vi "CPP-GRCserver.vi"(4 "minFlowrate (l/min)":dbl format="%.2f", 5 "Pressure channel":string, 6 "maxFlowrate (l/min)":dbl format="%.2f", 7 "Temperature channel":string, 8 "C:Dem(%)":dbl caption="C:Dem(%) (0)" min=0.0 max=100.0 step=1.0 format="%.2f", 9 "Gas Release System":string, 10 "Q[Total]:Dem(l/min)":dbl caption="Q[Total]:Dem(l/min) (0)" format="%.2f", 11 "Mode":T1=enum."Close All MFCs" caption="Mode (CloseAll)") -> (0 "errorString":string, 1 "infoString":string, 3 "watchChannels":string[](array[string]))   [LabVIEW 2021]
uses:
  Sub VI's/Gas management/CPP/AalborgServerModes.ctl
  Sub VI's/Gas management/CPP/AalborgServerData.ctl
  Sub VI's/Gas management/CPP/MFCdescription.ctl
  Sub VI's/Gas management/CPP/MFCcapability.ctl
  Sub VI's/Gas management/CPP/AalborgServerControlBus.ctl
  Sub VI's/Gas management/CPP/AalborgServerStates.ctl
  ADAM Client/Sub VIs/ADAM Controls/Channel_State.ctl
  ADAM Client/Sub VIs/ADAM Controls/Update_scan_value.ctl
  Anemometry/Anemometry Sub Vis/Controls/GasCombo.ctl
  f0e89fe8-b597-9c4c-bd9e-b7a5d13a6cec.vi
panel:
  in  "Tab Control":enum32{"I/O", "Control", "Data"}(tab)
  out "callNum":i32
  in  "idealSPFraction":dbl=0.95 format="%#_13g"
  out "Press:(mBar)":dbl
  out "Temp:(C)":dbl
  out "C2H6 massflow demand":dbl format="%#_g g/min"
  out "N2 massflow demand":dbl format="%#_g g/min"
  out "C2H6 flowrate demand":dbl format="%#_g l/min"
  out "N2 flowrate demand":dbl format="%#_g l/min"
  out "runTime(s)":dbl
  out "ControlBus":T2={"ActionPath"=[enum."ComputeFlowrates", enum."ADAMiseDemands", enum."ListMFCchannels", enum."ChooseMFCs", enum."CalculateSetpoints", enum."ExecuteSetpoints", enum."Summarise"], "step"=0, "Done?"=FALSE, "Messages"="", "deltaQ"=0.0, "deltaC"=0.0}
  out "DataBus":T4 {"RhoTrace" format="%.3gg/l"; "RhoCarrier" format="%.3gg/l"; "InactiveC2H6MFCs"."mDot" format="%_4g"; "InactiveC2H6MFCs"."Setpoint" format="%.2g"; "InactiveC2H6MFCs"."MFCcapability"."MaxMdot" format="%_4g"; "InactiveC2H6MFCs"."MFCcapability"."MinMdot" format="%_4g"; "ActiveC2H6MFCs"."mDot" format="%_4g"; "ActiveC2H6MFCs"."Setpoint" format="%.2g"; "ActiveC2H6MFCs"."MFCcapability"."MaxMdot" format="%_4g"; "ActiveC2H6MFCs"."MFCcapability"."MinMdot" format="%_4g"; "InactiveN2MFCs"."mDot" format="%_4g"; "InactiveN2MFCs"."Setpoint" format="%.2g"; "InactiveN2MFCs"."MFCcapability"."MaxMdot" format="%_4g"; "InactiveN2MFCs"."MFCcapability"."MinMdot" format="%_4g"; "ActiveN2MFCs"."mDot" format="%_4g"; "ActiveN2MFCs"."Setpoint" format="%.2g"; "ActiveN2MFCs"."MFCcapability"."MaxMdot" format="%_4g"; "ActiveN2MFCs"."MFCcapability"."MinMdot" format="%_4g"; "C2H6MFCs"."mDot" format="%_4g"; "C2H6MFCs"."Setpoint" format="%.2g"; "C2H6MFCs"."MFCcapability"."MaxMdot" format="%_4g"; "C2H6MFCs"."MFCcapability"."MinMdot" format="%_4g"; "N2MFCs"."mDot" format="%_4g"; "N2MFCs"."Setpoint" format="%.2g"; "N2MFCs"."MFCcapability"."MaxMdot" format="%_4g"; "N2MFCs"."MFCcapability"."MinMdot" format="%_4g"; "QdemCarrier" format="%.2pl/min"; "QdemTrace" format="%.2pl/min"; "MdotCarrier" format="%_4pg/min"; "MdotTrace" format="%_4pg/min"; "releaseTemp" format="%#_gC"; "releasePress" format="%#_gmBar"}
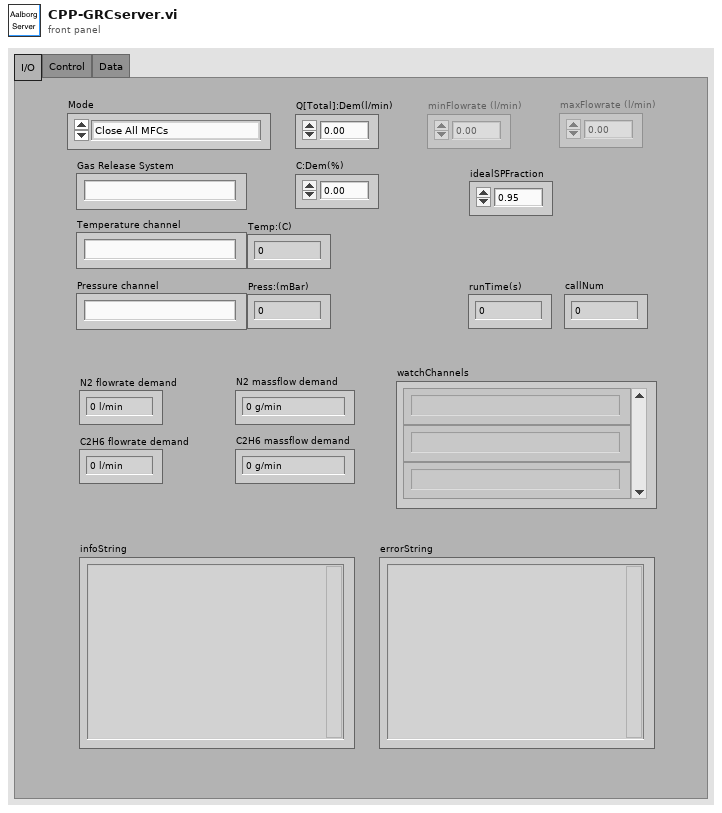
[diagram p1: front panel]
types:
  T1 = typedef "AalborgServerModes.ctl" = enum16{"Set Flows", "Check Flows Are Achievable", "Close All MFCs"}
  T2 = typedef "AalborgServerControlBus.ctl" = cluster{"ActionPath":T3[], "step":i32, "Done?":bool, "Messages":string, "deltaQ":dbl, "deltaC":dbl}
  T3 = typedef "AalborgServerStates.ctl" = enum16{"Initialise", "Supervise", "WhatNext", "ComputeFlowrates", "ADAMiseDemands", "ListMFCchannels", "ChooseMFCs", "CalculateSetpoints", "ExecuteSetpoints", "SetScanRates", "CloseAll", "Summarise"}
  T4 = typedef "AalborgServerData.ctl" = cluster{"releaseTemp":dbl, "releasePress":dbl, "QdemCarrier":dbl, "QdemTrace":dbl, "MdotCarrier":dbl, "MdotCarrierMin":dbl, "MdotCarrierMax":dbl, "MdotTrace":dbl, "MdotTraceMin":dbl, "MdotTraceMax":dbl, "N2MFCs":T5[], "C2H6MFCs":T5[], "CarrierOffIdeal":dbl, "TraceOffIdeal":dbl, "ActiveN2MFCs":T5[], "InactiveN2MFCs":T5[], "ActiveC2H6MFCs":T5[], "InactiveC2H6MFCs":T5[], "RhoCarrier":dbl, "RhoTrace":dbl}
  T5 = typedef "MFCdescription.ctl" = cluster{"BaseName":string, "MFCcalibration":cluster{"Y(100)":dbl, "Y(0)":dbl, "SPmin(%)":dbl, "SPmax(%)":dbl}, "MFCcapability":T6, "InUse?":bool, "Setpoint":dbl, "mDot":dbl}
  T6 = typedef "MFCcapability.ctl" = cluster{"Gas":string, "MinMdot":dbl, "MaxMdot":dbl}
  T7 = typedef "Channel_State.ctl" = enum16{"On", "Off", "Always On", "Always Off"}
  T8 = typedef "GasCombo.ctl" = string
  T9 = typedef "Update_scan_value.ctl" = cluster{"Channel Name":string, "New Value":dbl, "!Auto_Off":bool}
  T10 = typedef "Ch_description_ADAM.ctl" = cluster{"Ch Name":string, "Type":T11, "Function":T12, "Ch State":T7, "Calibration type":T13, "A":dbl, "B":dbl, "C":dbl, "D":dbl, "Comments":string, "Address":T14, "String":string, "Duty":u16}
  T11 = typedef "Module_type_ADAM.ctl" = string
  T12 = typedef "Function_ADAM.ctl" = enum16{"Analogue Input", "Digital Input", "Event counter", "Event rate", "Analogue Output", "Digital Output", "Relay Output"}
  T13 = typedef "Calib_type_ADAM.ctl" = string
  T14 = typedef "Address.ctl" = cluster{"Main":i32, "Ch.":i32, "Sub":i32, "Port Name":string}
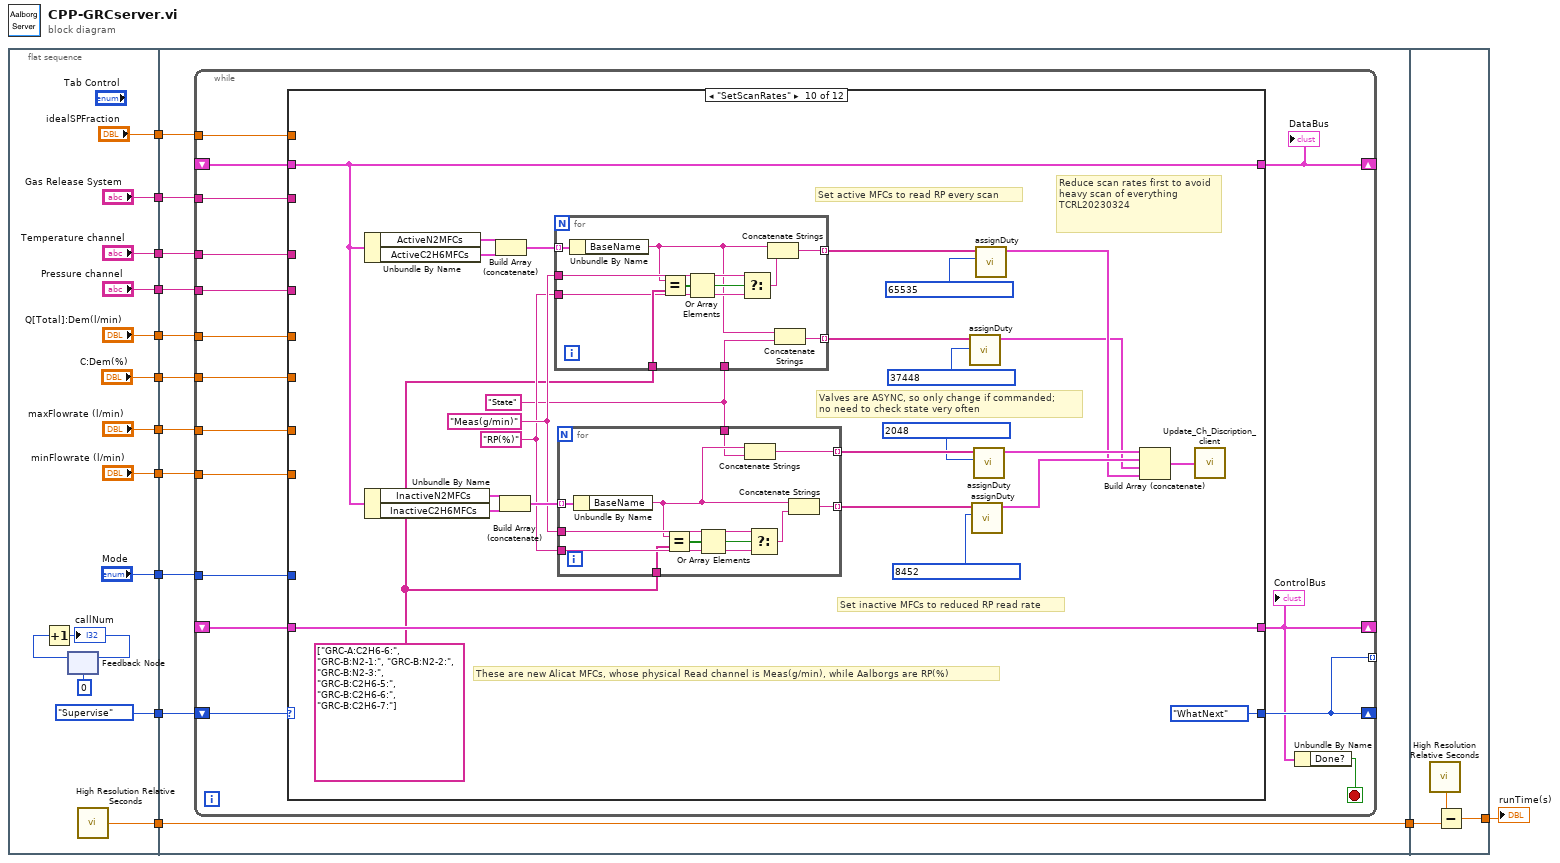
[diagram p0: block diagram]
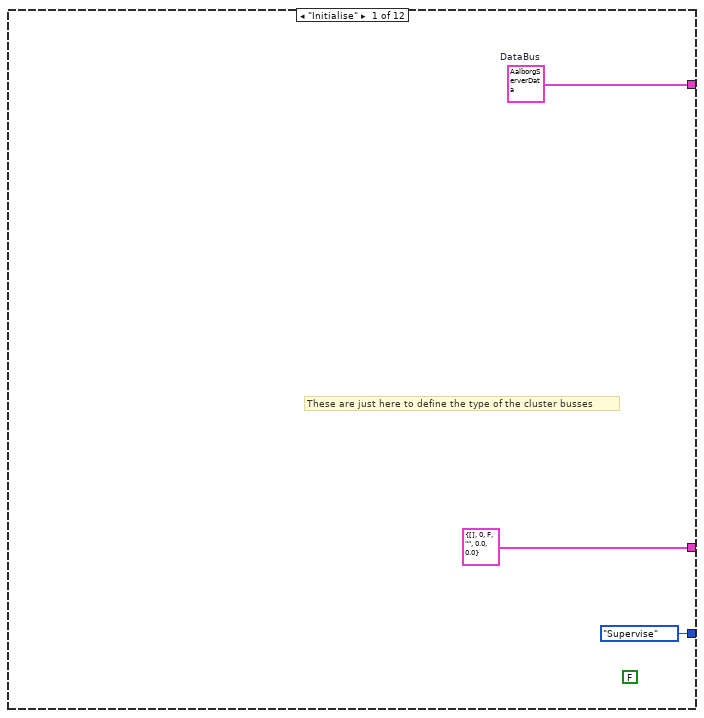
[diagram p2: hidden frame]
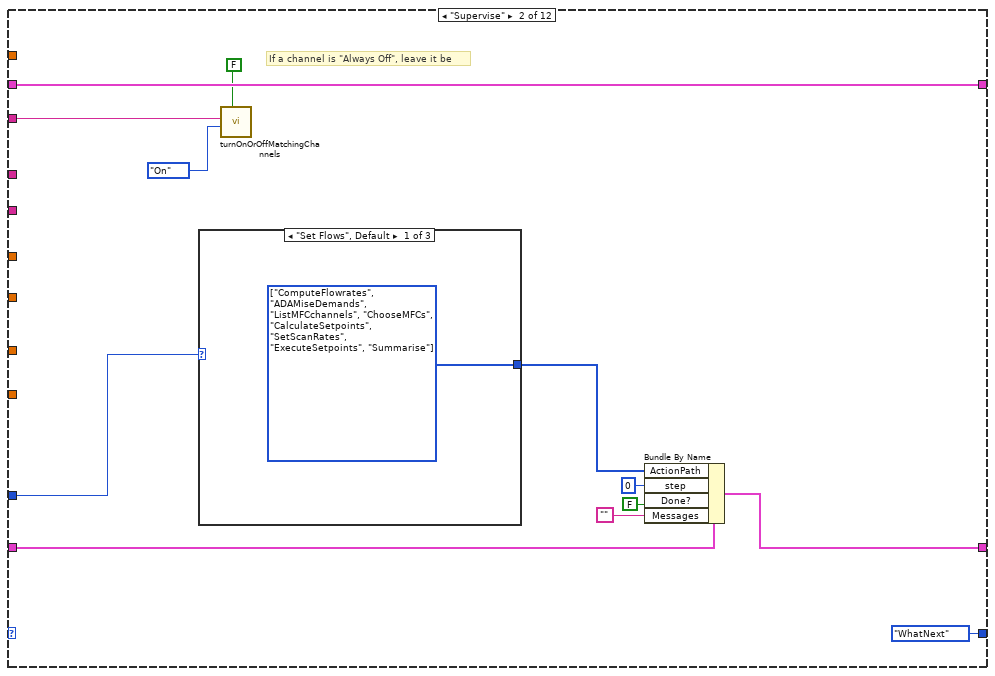
[diagram p3: hidden frame]
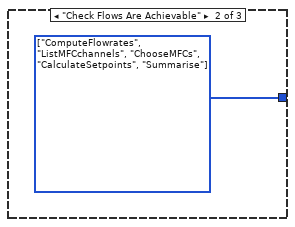
[diagram p4: hidden frame]
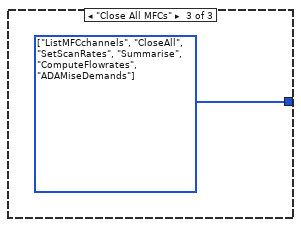
[diagram p5: hidden frame]
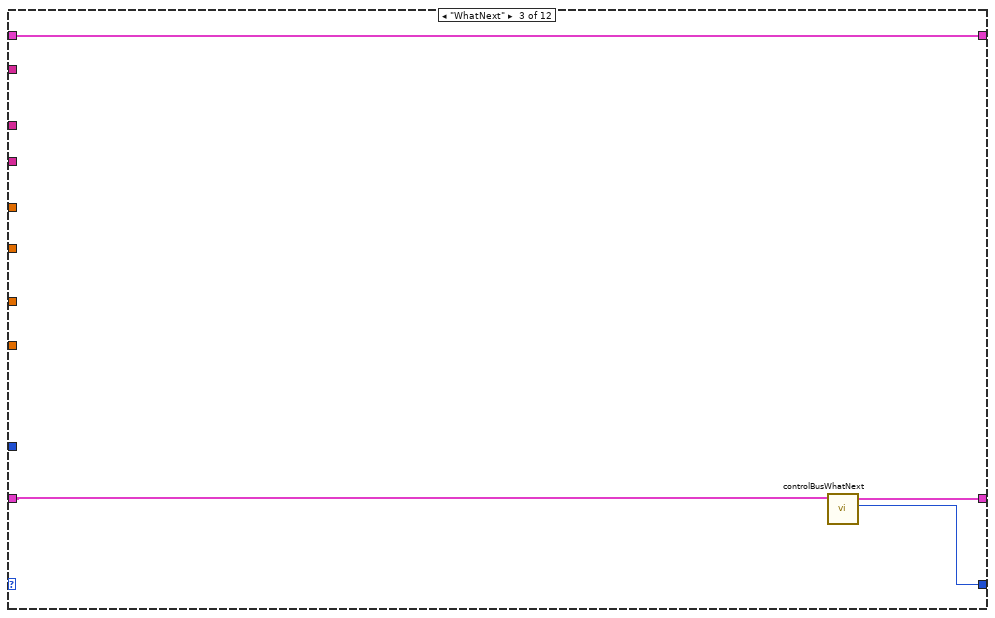
[diagram p6: hidden frame]
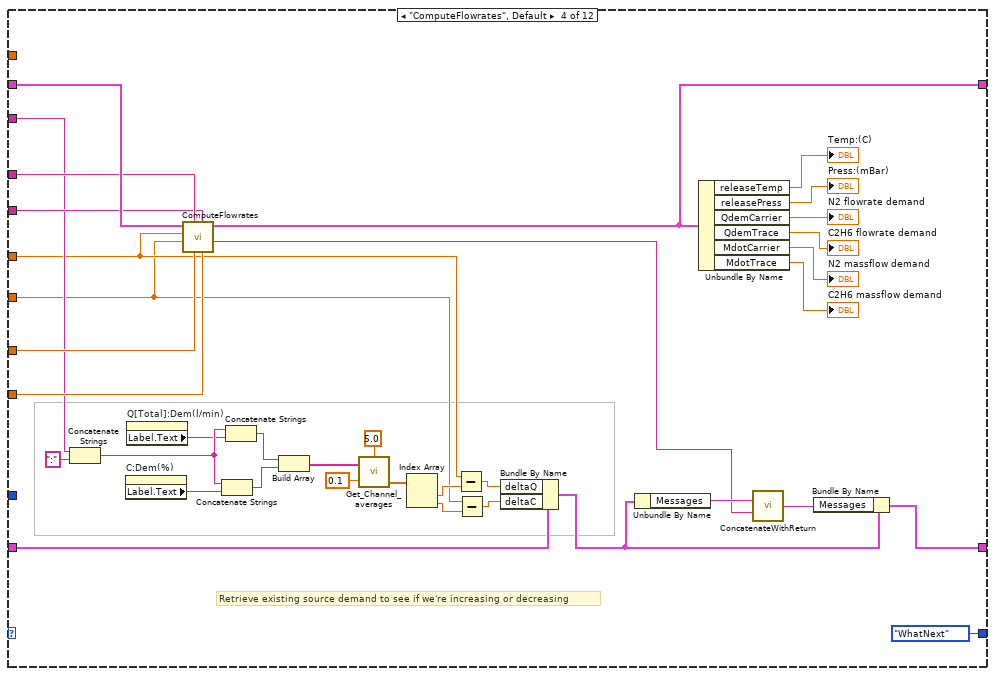
[diagram p7: hidden frame]
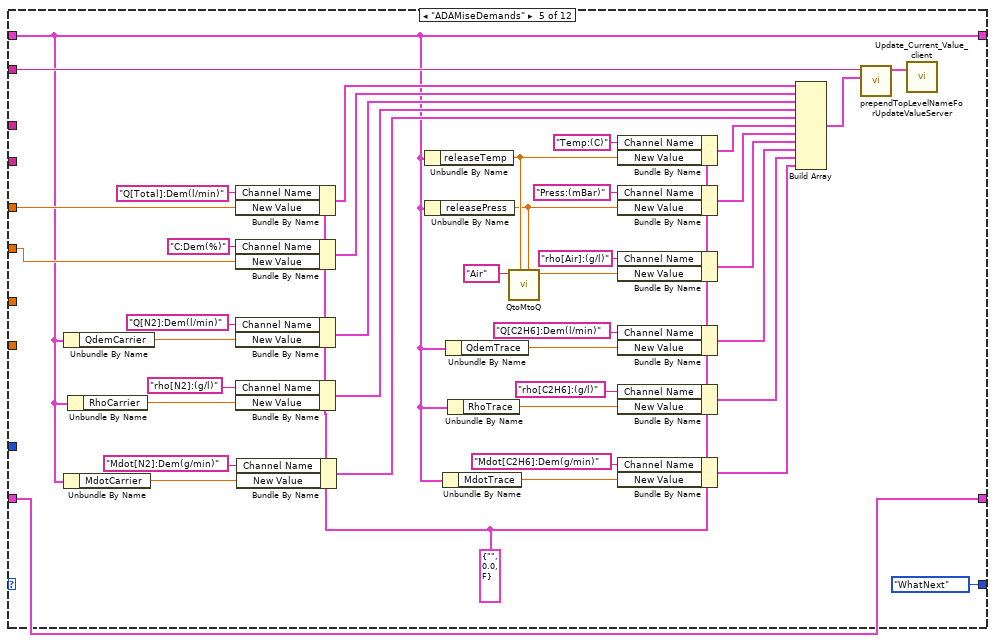
[diagram p8: hidden frame]
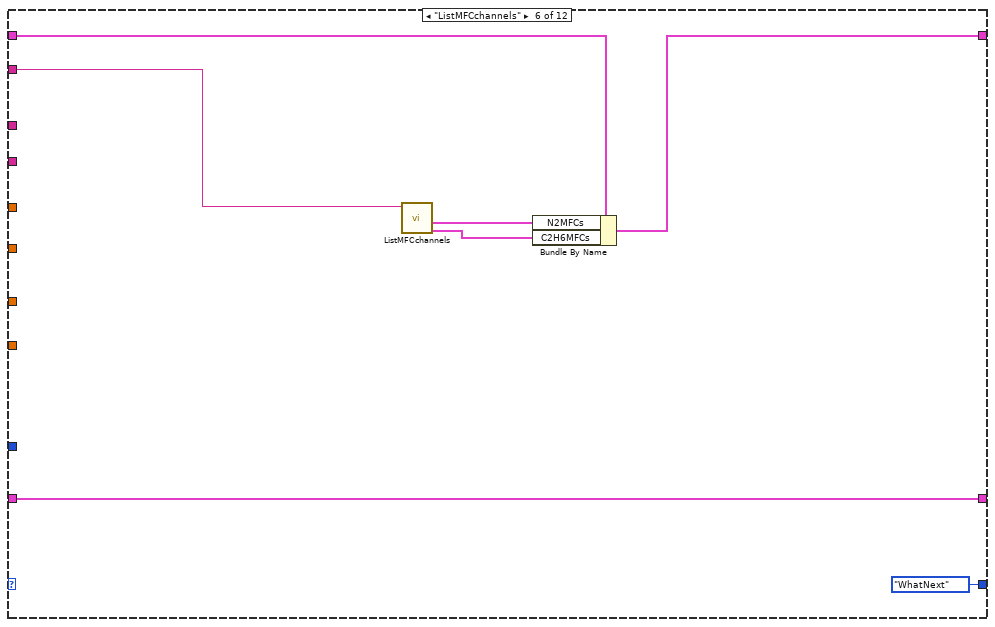
[diagram p9: hidden frame]
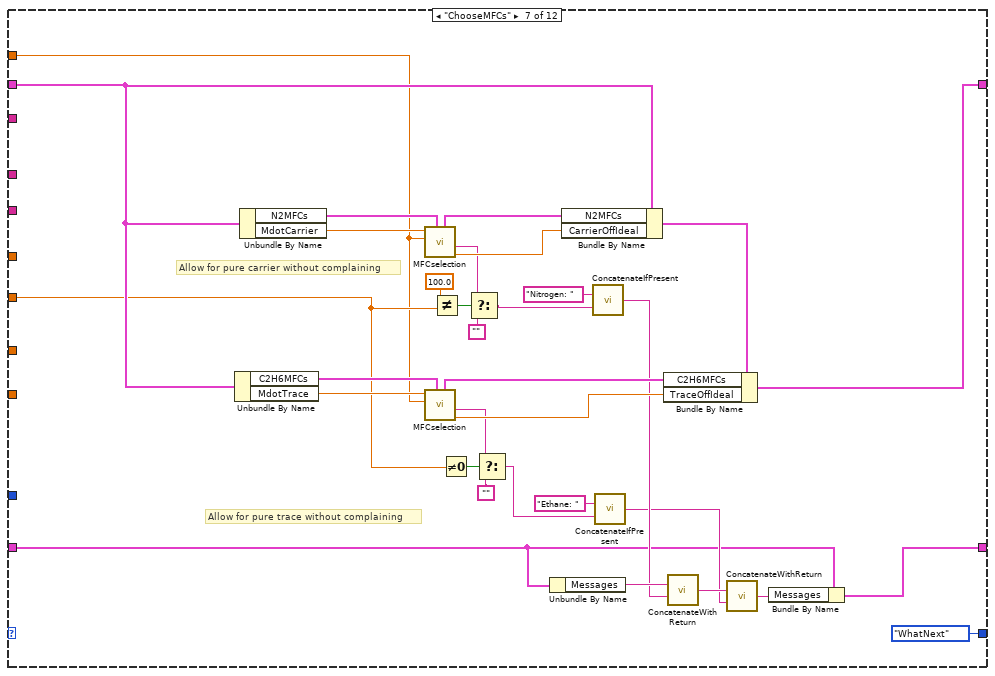
[diagram p10: hidden frame]
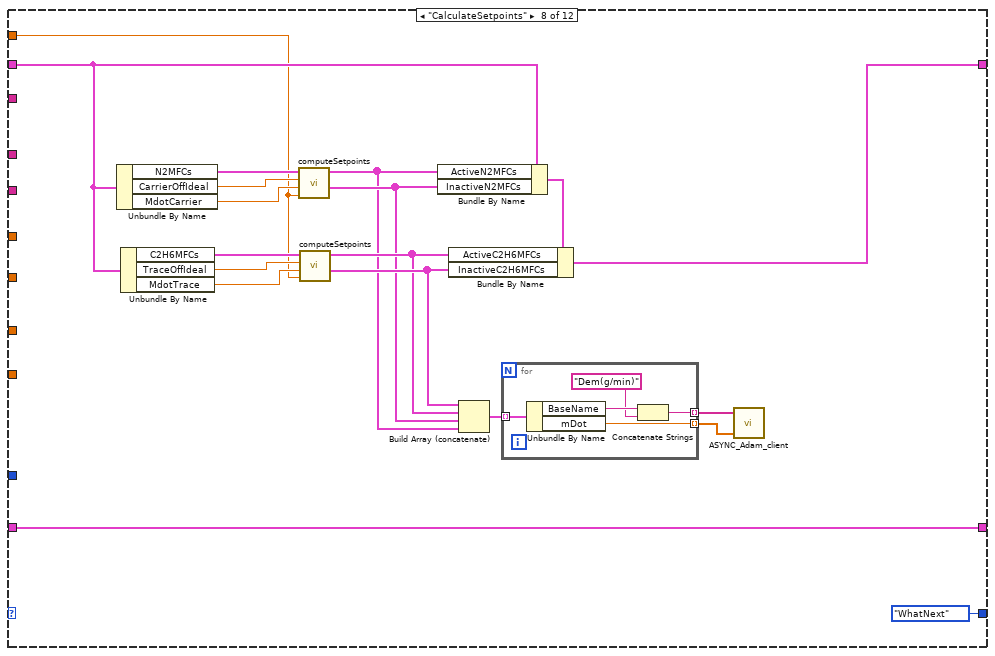
[diagram p11: hidden frame]
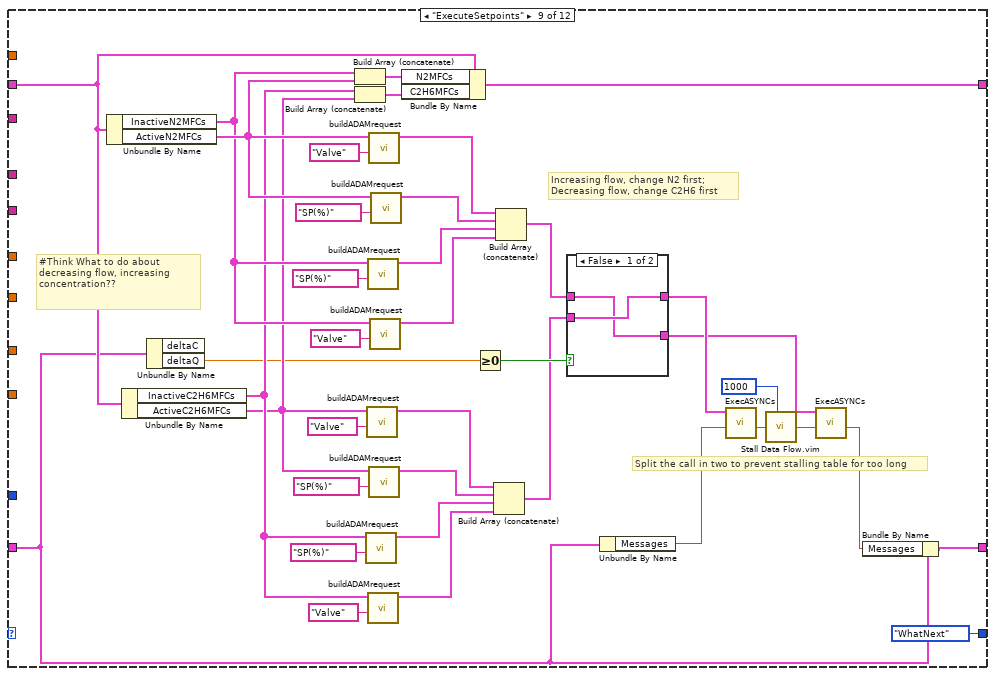
[diagram p12: hidden frame]
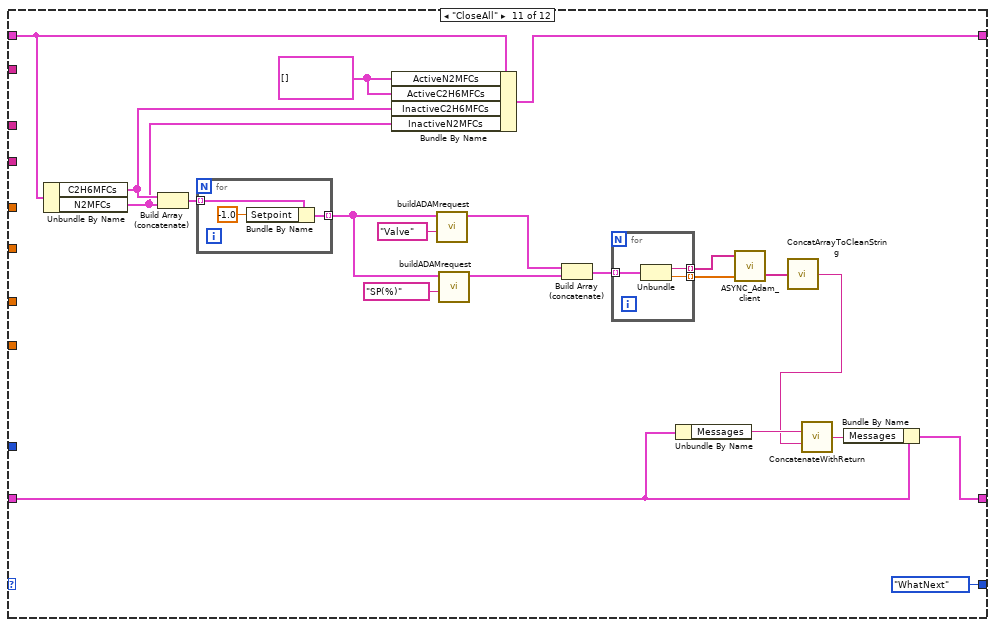
[diagram p14: hidden frame]
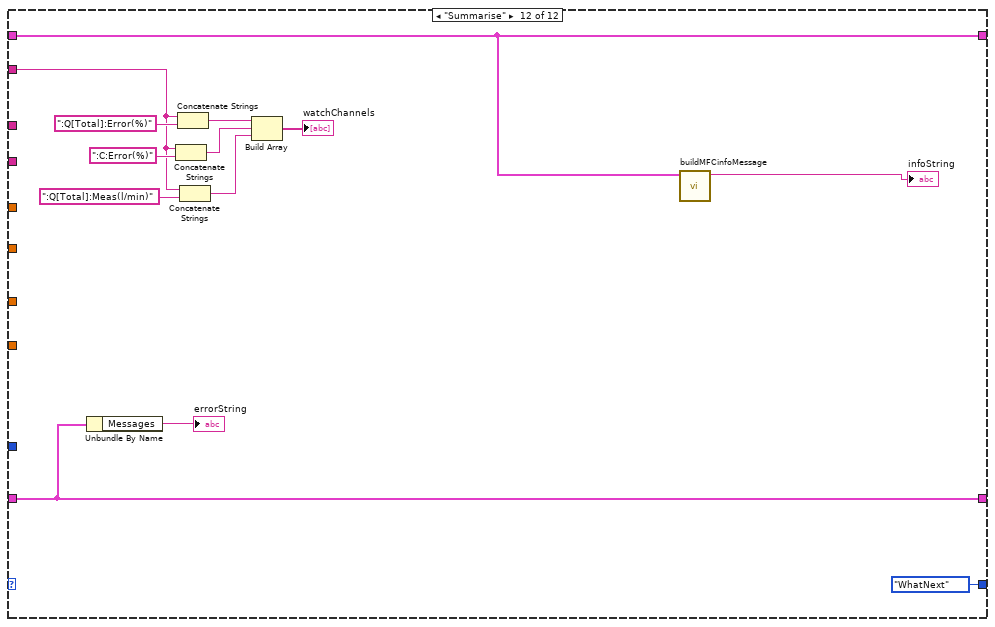
[diagram p15: hidden frame]
diagram:
  n1 = flat-sequence {
    tunnel: ["idealSPFraction"] -> w13
    tunnel: ["Gas Release System"] -> w12
    tunnel: ["Pressure channel"] -> w11
    tunnel: ["Temperature channel"] -> w10
    tunnel: ["C:Dem(%)"] -> w9
    tunnel: ["Q[Total]:Dem(l/min)"] -> w8
    tunnel: ["maxFlowrate (l/min)"] -> w7
    tunnel: ["minFlowrate (l/min)"] -> w6
    tunnel: ["Mode"] -> w5
    tunnel: [AalborgServerStates."Supervise"] -> w4
    tunnel: [w17] -> w2
    tunnel: w13 -> [w38]
    tunnel: w12 -> [w37]
    tunnel: w11 -> [w36]
    tunnel: w10 -> [w35]
    tunnel: w9 -> [w34]
    tunnel: w8 -> [w33]
    tunnel: w7 -> [w32]
    tunnel: w6 -> [w31]
    tunnel: w5 -> [w30]
    tunnel: w4 -> [w29]
    tunnel: [w28] -> w3
    tunnel: w2 -> [w28]
    tunnel: w3 -> [w348]
    tunnel: [w347] -> w1
    frame #0 {
      n2 = feedback #1(0) -> (w15:i32)
      n3 = Increment(x=w15) -> (x+1=w16:i32)
      "callNum" <- w16
      n4 = feedback-in #1(w16) -> ()
      n5 = call <vilib>:"High Resolution Relative Seconds.vi"() -> ("relative seconds"=w17:dbl)
    }
    frame #1 {
      n6 = while {
        shift-right: [w53] -> _
        shift-left: _ -> [w52]
        tunnel: w33 -> [w54]
        tunnel: w36 -> [w50]
        tunnel: w35 -> [w49]
        tunnel: w34 -> [w48]
        shift-right: [w42] -> _
        shift-left: w29 -> [w51]
        tunnel: w37 -> [w47]
        tunnel: w32 -> [w46]
        tunnel: w31 -> [w45]
        shift-right: [w40] -> _
        shift-left: _ -> [w41]
        tunnel: w30 -> [w44]
        tunnel: [w42] -> _ mode=indexing
        tunnel: w38 -> [w39]
        stop <- w43 stop-if-true
        n7 = case shown="\"SetScanRates\"" w51 {
          tunnel: w54 -> [_ _ _ w89 w145 _ _ _ _ _ _ _]
          tunnel: [w57 w69 w73 w85 w130 w158 w187 w201 w253 w278 w316 w339] -> w53
          tunnel: w52 -> [_ w69 w73 w112 w130 w159 w192 w203 w233 w278 w317 w339]
          tunnel: w50 -> [_ _ _ w110 _ _ _ _ _ _ _ _]
          tunnel: w49 -> [_ _ _ w111 _ _ _ _ _ _ _ _]
          tunnel: w48 -> [_ _ _ w87 w148 _ w174 _ _ _ _ _]
          tunnel: w47 -> [_ w59 _ w90 w147 w160 _ _ _ _ _ w335]
          tunnel: [AalborgServerStates."Supervise" AalborgServerStates."WhatNext" ("whereNext") w74 AalborgServerStates."WhatNext" ("whereNext") AalborgServerStates."WhatNext" ("whereNext") AalborgServerStates."WhatNext" ("whereNext") AalborgServerStates."WhatNext" ("whereNext") AalborgServerStates."WhatNext" ("whereNext") AalborgServerStates."WhatNext" ("whereNext") AalborgServerStates."WhatNext" ("whereNext") AalborgServerStates."WhatNext" ("whereNext") AalborgServerStates."WhatNext" ("whereNext")] -> w42
          tunnel: w46 -> [_ _ _ w103 _ _ _ _ _ _ _ _]
          tunnel: w45 -> [_ _ _ w102 _ _ _ _ _ _ _ _]
          tunnel: w41 -> [_ w67 w75 w82 w143 w155 w164 w208 w225 w274 w308 w344]
          tunnel: [T2 {"ActionPath"=[], "step"=0, "Done?"=FALSE, "Messages"="", "deltaQ"=0.0, "deltaC"=0.0} ("busOut") w65 w76 w77 w143 w155 w163 w208 w224 w274 w309 w344] -> w40
          tunnel: w44 -> [_ w68 _ _ _ _ _ _ _ _ _ _]
          tunnel: w39 -> [_ _ _ _ _ _ w161 w193 _ _ _ _]
          frame "Initialise" {
            (unwired) FALSE
            w57 = T4 {"releaseTemp"=0.0, "releasePress"=0.0, "QdemCarrier"=0.0, "QdemTrace"=0.0, "MdotCarrier"=0.0, "MdotCarrierMin"=0.0, "MdotCarrierMax"=0.0, "MdotTrace"=0.0, "MdotTraceMin"=0.0, "MdotTraceMax"=0.0, "N2MFCs"=[], "C2H6MFCs"=[], "CarrierOffIdeal"=0.0, "TraceOffIdeal"=0.0, "ActiveN2MFCs"=[], "InactiveN2MFCs"=[], "ActiveC2H6MFCs"=[], "InactiveC2H6MFCs"=[], "RhoCarrier"=0.0, "RhoTrace"=0.0}  # DataBus
            # "These are just here to define the type of the cluster busses"
          }
          frame "Supervise" {
            # "If a channel is \"Always Off\", leave it be"
            n8 = case shown="\"Set Flows\", Default" w68 {
              tunnel: [w70 w71 w72] -> w66
              frame "Set Flows", Default {
                w70 = T3[] [enum."ComputeFlowrates", enum."ADAMiseDemands", enum."ListMFCchannels", enum."ChooseMFCs", enum."CalculateSetpoints", enum."SetScanRates", enum."ExecuteSetpoints", enum."Summarise"] items=["Initialise", "Supervise", "WhatNext", "ComputeFlowrates", "ADAMiseDemands", "ListMFCchannels", "ChooseMFCs", "CalculateSetpoints", "ExecuteSetpoints", "SetScanRates", "CloseAll", "Summarise"]
              }
              frame "Check Flows Are Achievable" {
                w71 = T3[] [enum."ComputeFlowrates", enum."ListMFCchannels", enum."ChooseMFCs", enum."CalculateSetpoints", enum."Summarise"] items=["Initialise", "Supervise", "WhatNext", "ComputeFlowrates", "ADAMiseDemands", "ListMFCchannels", "ChooseMFCs", "CalculateSetpoints", "ExecuteSetpoints", "SetScanRates", "CloseAll", "Summarise"]
              }
              frame "Close All MFCs" {
                w72 = T3[] [enum."ListMFCchannels", enum."CloseAll", enum."SetScanRates", enum."Summarise", enum."ComputeFlowrates", enum."ADAMiseDemands"] items=["Initialise", "Supervise", "WhatNext", "ComputeFlowrates", "ADAMiseDemands", "ListMFCchannels", "ChooseMFCs", "CalculateSetpoints", "ExecuteSetpoints", "SetScanRates", "CloseAll", "Summarise"]
              }
            }
            n9 = call "turnOnOrOffMatchingChannels.vi"("override\"Always\"chs"=FALSE ("override\"Always\"chs"), "setState"=Channel_State."On", "regular expression"=w59) -> ()  [unwired: 6 in, 3 out]
            n10 = Bundle By Name(cluster=w67, "ActionPath"=w66, "step"=0, "Done?"=FALSE, "Messages"="") -> (w65:T2)
          }
          frame "WhatNext" {
            n11 = call "controlBusWhatNext.vi"("busIn"=w75) -> ("whereNext"=w74:T3, "busOut"=w76:T2)  [unwired: 9 in]
          }
          frame "ComputeFlowrates", Default {
            # "Retrieve existing source demand to see if we're increasing or decreasing"
            n12 = Concatenate Strings(w90, ":" ("string")) -> (w92:string)
            n13 = property on="C:Dem(%)" class="DigNum (strict)"() -> ("Label.Text"=w96:string)  [unwired: 2 in, 2 out]
            n14 = property on="Q[Total]:Dem(l/min)" class="DigNum (strict)"() -> ("Label.Text"=w91:string)  [unwired: 2 in, 2 out]
            n15 = call "ComputeFlowrates.vi"("minFlowrate (l/min)"=w102, "Pressure channel"=w110, "maxFlowrate (l/min)"=w103, "Temperature channel"=w111, "C_dem:(%)"=w87, "Q_dem[Total]:(l/min)"=w89, "DataBus in"=w112) -> ("errorString"=w80:string, "DataBus out"=w85:T4)  [unwired: 3 in]
            n16 = Concatenate Strings(w92, w96) -> (w94:string)
            n17 = Concatenate Strings(w92, w91) -> (w95:string)
            n18 = Build Array(w95, w94) -> (w97:string[])
            n19 = call "Get_Channel_averages.vi"("Desired Ch Names"=w97, "Averaging time (mins)"=0.1, "End Offset Sec (0)"=5.0) -> ("number"=w100:dbl[])  [unwired: 2 out]
            n20 = Index Array(array=w100) -> (element #1=w88:dbl, element #2=w86:dbl)  [unwired: 2 in]
            n21 = Subtract(x=w89, y=w88) -> (x-y=w84:dbl)
            n22 = Subtract(x=w87, y=w86) -> (x-y=w83:dbl)
            n23 = Bundle By Name(cluster=w82, "deltaQ"=w84, "deltaC"=w83) -> (w78:T2)
            n24 = Unbundle By Name(w78) -> ("Messages"=w81:string)
            n25 = Unbundle By Name(w85) -> ("releaseTemp"=→"Temp:(C)":dbl, "releasePress"=→"Press:(mBar)":dbl, "QdemCarrier"=→"N2 flowrate demand":dbl, "QdemTrace"=→"C2H6 flowrate demand":dbl, "MdotCarrier"=→"N2 massflow demand":dbl, "MdotTrace"=→"C2H6 massflow demand":dbl)
            n26 = call "ConcatenateWithReturn.vi"("baseString"=w81, "additionalString"=w80) -> ("outputString"=w79:string)  [unwired: 13 in]
            n27 = Bundle By Name(cluster=w78, "Messages"=w79) -> (w77:T2)
          }
          frame "ADAMiseDemands" {
            w116 = T9 {"Channel Name"="", "New Value"=0.0, "!Auto_Off"=FALSE} ("Update Scan Value Cluster")
            n28 = Unbundle By Name(w130) -> ("QdemCarrier"=w152:dbl)
            n29 = Unbundle By Name(w130) -> ("MdotCarrier"=w150:dbl)
            n30 = Unbundle By Name(w130) -> ("RhoCarrier"=w146:dbl)
            n31 = Bundle By Name(cluster=w116, "Channel Name"="Q[Total]:Dem(l/min)", "New Value"=w145) -> (w140:T9)
            n32 = Bundle By Name(cluster=w116, "Channel Name"="C:Dem(%)", "New Value"=w148) -> (w139:T9)
            n33 = Bundle By Name(cluster=w116, "Channel Name"="Q[N2]:Dem(l/min)", "New Value"=w152) -> (w138:T9)
            n34 = Bundle By Name(cluster=w116, "Channel Name"="rho[N2]:(g/l)", "New Value"=w146) -> (w137:T9)
            n35 = Bundle By Name(cluster=w116, "Channel Name"="Mdot[N2]:Dem(g/min)", "New Value"=w150) -> (w136:T9)
            n36 = Unbundle By Name(w130) -> ("releaseTemp"=w119:dbl)
            n37 = Unbundle By Name(w130) -> ("releasePress"=w118:dbl)
            n38 = Unbundle By Name(w130) -> ("MdotTrace"=w149:dbl)
            n39 = Unbundle By Name(w130) -> ("QdemTrace"=w151:dbl)
            n40 = Unbundle By Name(w130) -> ("RhoTrace"=w142:dbl)
            n41 = call "QtoMtoQ.vi"("Pressure"=w118, "Temperature"=w119, "Gas"=T8 "Air") -> ("Density (kg/m^3)(= g/l)"=w115:dbl)  [unwired: 4 in, 2 out]
            n42 = Bundle By Name(cluster=w116, "Channel Name"="Temp:(C)", "New Value"=w119) -> (w135:T9)
            n43 = Bundle By Name(cluster=w116, "Channel Name"="Press:(mBar)", "New Value"=w118) -> (w134:T9)
            n44 = Bundle By Name(cluster=w116, "Channel Name"="rho[Air]:(g/l)", "New Value"=w115) -> (w113:T9)
            n45 = Bundle By Name(cluster=w116, "Channel Name"="Q[C2H6]:Dem(l/min)", "New Value"=w151) -> (w133:T9)
            n46 = Bundle By Name(cluster=w116, "Channel Name"="rho[C2H6]:(g/l)", "New Value"=w142) -> (w132:T9)
            n47 = Bundle By Name(cluster=w116, "Channel Name"="Mdot[C2H6]:Dem(g/min)", "New Value"=w149) -> (w131:T9)
            n48 = Build Array(w140, w139, w138, w137, w136, w135, w134, w113, w133, w132, w131) -> (w141:T9[])
            n49 = call "prependTopLevelNameForUpdateValueServer.vi"("Array in"=w141, "TopLevelADAMname"=w147) -> ("Array out"=w153:T9[])  [unwired: 9 in]
            n50 = call "Update_Current_Value_client.vi"("Update array in"=w153) -> ()  [unwired: 1 in]
          }
          frame "ListMFCchannels" {
            n51 = call "ListMFCchannels.vi"("Gas Release System"=w160) -> ("C2H6descriptions"=w156:T5[], "N2descriptions"=w157:T5[])  [unwired: 9 in]
            n52 = Bundle By Name(cluster=w159, "N2MFCs"=w157, "C2H6MFCs"=w156) -> (w158:T4)
          }
          frame "ChooseMFCs" {
            # "Allow for pure carrier without complaining"
            # "Allow for pure trace without complaining"
            n53 = Unbundle By Name(w192) -> ("C2H6MFCs"=w186:T5[], "MdotTrace"=w181:dbl)
            n54 = Unbundle By Name(w192) -> ("N2MFCs"=w183:T5[], "MdotCarrier"=w182:dbl)
            n55 = call "MFCselection.vi"("MFCsIn"=w183, "idealSPFraction"=w161, "Mdot"=w182) -> ("OffIdeal"=w185:dbl, "errorReport"=w171:string, "MFCsOut"=w184:T5[])  [unwired: 3 in, 1 out]
            n56 = call "MFCselection.vi"("MFCsIn"=w186, "idealSPFraction"=w161, "Mdot"=w181) -> ("OffIdeal"=w189:dbl, "errorReport"=w179:string, "MFCsOut"=w190:T5[])  [unwired: 3 in, 1 out]
            n57 = Not Equal?(x=100.0, y=w174) -> (x != y?=w170:bool)
            n58 = Not Equal To 0?(x=w174) -> (x != 0?=w180:bool)
            n59 = Select(t=w171, s=w170, f="") -> (s? t:f=w172:string)
            n60 = Select(t=w179, s=w180, f="") -> (s? t:f=w175:string)
            n61 = Unbundle By Name(w164) -> ("Messages"=w168:string)
            n62 = Bundle By Name(cluster=w192, "N2MFCs"=w184, "CarrierOffIdeal"=w185) -> (w188:T4)
            n63 = call "ConcatenateIfPresent.vi"("prependString"="Nitrogen: ", "appendString"=w172) -> ("outputString"=w167:string)  [unwired: 13 in]
            n64 = call "ConcatenateIfPresent.vi"("prependString"="Ethane: ", "appendString"=w175) -> ("outputString"=w165:string)  [unwired: 13 in]
            n65 = Bundle By Name(cluster=w188, "C2H6MFCs"=w190, "TraceOffIdeal"=w189) -> (w187:T4)
            n66 = call "ConcatenateWithReturn.vi"("baseString"=w168, "additionalString"=w167) -> ("outputString"=w166:string)  [unwired: 13 in]
            n67 = call "ConcatenateWithReturn.vi"("baseString"=w166, "additionalString"=w165) -> ("outputString"=w162:string)  [unwired: 13 in]
            n68 = Bundle By Name(cluster=w164, "Messages"=w162) -> (w163:T2)
          }
          frame "CalculateSetpoints" {
            n69 = Unbundle By Name(w203) -> ("N2MFCs"=w209:T5[], "CarrierOffIdeal"=w211:dbl, "MdotCarrier"=w210:dbl)
            n70 = Unbundle By Name(w203) -> ("C2H6MFCs"=w206:T5[], "TraceOffIdeal"=w204:dbl, "MdotTrace"=w205:dbl)
            n71 = call "computeSetpoints.vi"("idealSPFraction"=w193, "Mdot"=w210, "OffIdeal"=w211, "MFCsIn"=w209) -> ("InactiveMFCs 2"=w195:T5[], "ActiveMFCs"=w194:T5[])  [unwired: 6 in]
            n72 = call "computeSetpoints.vi"("idealSPFraction"=w193, "Mdot"=w205, "OffIdeal"=w204, "MFCsIn"=w206) -> ("InactiveMFCs 2"=w197:T5[], "ActiveMFCs"=w196:T5[])  [unwired: 6 in]
            n73 = Bundle By Name(cluster=w203, "ActiveN2MFCs"=w194, "InactiveN2MFCs"=w195) -> (w202:T4)
            n74 = Bundle By Name(cluster=w202, "ActiveC2H6MFCs"=w196, "InactiveC2H6MFCs"=w197) -> (w201:T4)
            n75 = Build Array (concatenate)(w197, w196, w195, w194) -> (w200:T5[])
            n76 = for {
              tunnel: w200 -> [w216] mode=indexing
              tunnel: [w213] -> w199 mode=indexing
              tunnel: [w212] -> w198 mode=indexing
              n77 = Unbundle By Name(w216) -> ("BaseName"=w215:string, "mDot"=w212:dbl)
              n78 = Concatenate Strings(w215, "Dem(g/min)" ("string")) -> (w213:string)
            }
            n79 = call "ASYNC_Adam_client.vi"("Values"=w198, "Channel Names"=w199) -> ()  [unwired: 1 in, 2 out]
          }
          frame "ExecuteSetpoints" {
            # "Split the call in two to prevent stalling table for too long"
            # "#Think What to do about decreasing flow, increasing concentration??"
            # "Increasing flow, change N2 first;\nDecreasing flow, change C2H6 first"
            n80 = Unbundle By Name(w233) -> ("InactiveN2MFCs"=w247:T5[], "ActiveN2MFCs"=w250:T5[])
            n81 = Unbundle By Name(w233) -> ("InactiveC2H6MFCs"=w228:T5[], "ActiveC2H6MFCs"=w227:T5[])
            n82 = Unbundle By Name(w225) -> ("deltaQ"=w226:dbl)  [unwired: 1 out]
            n83 = Build Array (concatenate)(w247, w250) -> (w254:T5[])
            n84 = Build Array (concatenate)(w228, w227) -> (w229:T5[])
            n85 = call "buildADAMrequest.vi"("Aspect"="SP(%)", "MFCs"=w228) -> ("ADAMrequests"=w240:cluster{"String":string, "Setpoint":dbl}[])  [unwired: 9 in]
            n86 = call "buildADAMrequest.vi"("Aspect"="Valve", "MFCs"=w227) -> ("ADAMrequests"=w238:cluster{"String":string, "Setpoint":dbl}[])  [unwired: 9 in]
            n87 = call "buildADAMrequest.vi"("Aspect"="SP(%)", "MFCs"=w247) -> ("ADAMrequests"=w244:cluster{"String":string, "Setpoint":dbl}[])  [unwired: 9 in]
            n88 = call "buildADAMrequest.vi"("Aspect"="Valve", "MFCs"=w228) -> ("ADAMrequests"=w241:cluster{"String":string, "Setpoint":dbl}[])  [unwired: 9 in]
            n89 = call "buildADAMrequest.vi"("Aspect"="Valve", "MFCs"=w250) -> ("ADAMrequests"=w246:cluster{"String":string, "Setpoint":dbl}[])  [unwired: 9 in]
            n90 = call "buildADAMrequest.vi"("Aspect"="SP(%)", "MFCs"=w227) -> ("ADAMrequests"=w239:cluster{"String":string, "Setpoint":dbl}[])  [unwired: 9 in]
            n91 = call "buildADAMrequest.vi"("Aspect"="Valve", "MFCs"=w247) -> ("ADAMrequests"=w243:cluster{"String":string, "Setpoint":dbl}[])  [unwired: 9 in]
            n92 = call "buildADAMrequest.vi"("Aspect"="SP(%)", "MFCs"=w250) -> ("ADAMrequests"=w245:cluster{"String":string, "Setpoint":dbl}[])  [unwired: 9 in]
            n93 = Bundle By Name(cluster=w233, "N2MFCs"=w254, "C2H6MFCs"=w229) -> (w253:T4)
            n94 = Greater Or Equal To 0?(x=w226) -> (x >= 0?=w232:bool)
            n95 = Build Array (concatenate)(w238, w239, w240, w241) -> (w230:cluster{"String":string, "Setpoint":dbl}[])
            n96 = Build Array (concatenate)(w246, w245, w244, w243) -> (w231:cluster{"String":string, "Setpoint":dbl}[])
            n97 = case shown="False" w232 {
              tunnel: w231 -> [w255 w258]
              tunnel: w230 -> [w256 w257]
              tunnel: [w256 w258] -> w220
              tunnel: [w255 w257] -> w219
              frame False {
              }
              frame True {
              }
            }
            n98 = Unbundle By Name(w225) -> ("Messages"=w223:string)
            n99 = call "ExecASYNCs.vi"("messageIn"=w223, "nameValueArray"=w220) -> ("messageOut"=w222:string)  [unwired: 9 in]
            n100 = call "Stall Data Flow.vim"("value in"=w222, "milliseconds to wait"=u32 1000) -> ("value out"=w218:string)  [unwired: 1 out]
            n101 = call "ExecASYNCs.vi"("messageIn"=w218, "nameValueArray"=w219) -> ("messageOut"=w221:string)  [unwired: 9 in]
            n102 = Bundle By Name(cluster=w225, "Messages"=w221) -> (w224:T2)
          }
          frame "SetScanRates" {
            (unwired) u16 65535 ("Duty")
            w269 = "State" ("string")
            w259 = string[] ["GRC-A:C2H6-6:", "GRC-B:N2-1:", "GRC-B:N2-2:", "GRC-B:N2-3:", "GRC-B:C2H6-5:", "GRC-B:C2H6-6:", "GRC-B:C2H6-7:"]
            w272 = "Meas(g/min)" ("string")
            w271 = "RP(%)" ("string")
            # "These are new Alicat MFCs, whose physical Read channel is Meas(g/min), while Aalborgs are RP(%)"
            # "Valves are ASYNC, so only change if commanded;\nno need to check state very often"
            # "Reduce scan rates first to avoid heavy scan of everything\nTCRL20230324"
            # "Set inactive MFCs to reduced RP read rate"
            # "Set active MFCs to read RP every scan"
            n103 = Unbundle By Name(w278) -> ("ActiveN2MFCs"=w284:T5[], "ActiveC2H6MFCs"=w283:T5[])
            n104 = Unbundle By Name(w278) -> ("InactiveN2MFCs"=w279:T5[], "InactiveC2H6MFCs"=w280:T5[])
            n105 = Build Array (concatenate)(w284, w283) -> (w282:T5[])
            n106 = Build Array (concatenate)(w279, w280) -> (w281:T5[])
            n107 = for {
              tunnel: w282 -> [w306] mode=indexing
              tunnel: [w297] -> w268 mode=indexing
              tunnel: w259 -> [w305]
              tunnel: w272 -> [w303]
              tunnel: w271 -> [w302]
              tunnel: w269 -> [w298]
              tunnel: [w296] -> w263 mode=indexing
              n108 = Unbundle By Name(w306) -> ("BaseName"=w299:string)
              n109 = Equal?(x=w299, y=w305) -> (x = y?=w304:bool[])
              n110 = Or Array Elements(Boolean array=w304) -> (logical OR=w300:bool)
              n111 = Select(t=w303, s=w300, f=w302) -> (s? t:f=w301:string)
              n112 = Concatenate Strings(w299, w301) -> (w297:string)
              n113 = Concatenate Strings(w299, w298) -> (w296:string)
            }
            n114 = for {
              tunnel: w281 -> [w295] mode=indexing
              tunnel: [w294] -> w273 mode=indexing
              tunnel: w272 -> [w291]
              tunnel: w271 -> [w290]
              tunnel: w259 -> [w289]
              tunnel: w269 -> [w286]
              tunnel: [w285] -> w266 mode=indexing
              n115 = Unbundle By Name(w295) -> ("BaseName"=w287:string)
              n116 = Equal?(x=w287, y=w289) -> (x = y?=w293:bool[])
              n117 = Or Array Elements(Boolean array=w293) -> (logical OR=w288:bool)
              n118 = Concatenate Strings(w287, w286) -> (w285:string)
              n119 = Select(t=w291, s=w288, f=w290) -> (s? t:f=w292:string)
              n120 = Concatenate Strings(w287, w292) -> (w294:string)
            }
            n121 = call "assignDuty.vi"("Duty"=u16 37448, "Array in"=w263) -> ("Array out"=w260:T10[])  [unwired: 9 in]
            n122 = call "assignDuty.vi"("Duty"=u16 8452, "Array in"=w273) -> ("Array out"=w270:T10[])  [unwired: 9 in]
            n123 = call "assignDuty.vi"("Duty"=u16 2048, "Array in"=w266) -> ("Array out"=w265:T10[])  [unwired: 9 in]
            n124 = call "assignDuty.vi"("Duty"=u16 65535, "Array in"=w268) -> ("Array out"=w261:T10[])  [unwired: 9 in]
            n125 = Build Array (concatenate)(w265, w270, w260, w261) -> (w276:T10[])
            n126 = call "Update_Ch_Discription_client.vi"("Channels to update In"=w276) -> ()  [unwired: 1 out]
          }
          frame "CloseAll" {
            w313 = T5[] [] ("ActiveN2MFCs")
            n127 = Unbundle By Name(w317) -> ("C2H6MFCs"=w315:T5[], "N2MFCs"=w314:T5[])
            n128 = Build Array (concatenate)(w315, w314) -> (w321:T5[])
            n129 = for {
              tunnel: w321 -> [w330] mode=indexing
              tunnel: [w328] -> w322 mode=indexing
              n130 = Bundle By Name(cluster=w330, "Setpoint"=-1.0) -> (w328:T5)
            }
            n131 = Bundle By Name(cluster=w317, "ActiveN2MFCs"=w313, "ActiveC2H6MFCs"=w313, "InactiveC2H6MFCs"=w315, "InactiveN2MFCs"=w314) -> (w316:T4)
            n132 = call "buildADAMrequest.vi"("Aspect"="Valve", "MFCs"=w322) -> ("ADAMrequests"=w325:cluster{"String":string, "Setpoint":dbl}[])  [unwired: 9 in]
            n133 = call "buildADAMrequest.vi"("Aspect"="SP(%)", "MFCs"=w322) -> ("ADAMrequests"=w324:cluster{"String":string, "Setpoint":dbl}[])  [unwired: 9 in]
            n134 = Build Array (concatenate)(w325, w324) -> (w323:cluster{"String":string, "Setpoint":dbl}[])
            n135 = for {
              tunnel: w323 -> [w333] mode=indexing
              tunnel: [w332] -> w319 mode=indexing
              tunnel: [w331] -> w318 mode=indexing
              n136 = Unbundle(w333) -> ("String"=w332:string, "Setpoint"=w331:dbl)
            }
            n137 = Unbundle By Name(w308) -> ("Messages"=w311:string)
            n138 = call "ASYNC_Adam_client.vi"("Values"=w318, "Channel Names"=w319) -> ("Scan Comments"=w312:string[])  [unwired: 1 in, 1 out]
            n139 = call "ConcatArrayToCleanString.vi"("stringArray"=w312) -> ("cleanDelimitedString"=w307:string)  [unwired: 1 in]
            n140 = call "ConcatenateWithReturn.vi"("baseString"=w311, "additionalString"=w307) -> ("outputString"=w310:string)  [unwired: 13 in]
            n141 = Bundle By Name(cluster=w308, "Messages"=w310) -> (w309:T2)
          }
          frame "Summarise" {
            n142 = Unbundle By Name(w344) -> ("Messages"=→"errorString":string)
            n143 = Concatenate Strings(w335, ":C:Error(%)") -> (w336:string)
            n144 = Concatenate Strings(w335, ":Q[Total]:Error(%)") -> (w341:string)
            n145 = Concatenate Strings(w335, ":Q[Total]:Meas(l/min)") -> (w334:string)
            n146 = Build Array(w341, w336, w334) -> (→"watchChannels":string[])
            n147 = call "buildMFCinfoMessage.vi"("DataBus in"=w339) -> ("infoString"=→"infoString":string)  [unwired: 10 in]
          }
        }
        "DataBus" <- w53
        "ControlBus" <- w40
        n148 = Unbundle By Name(w40) -> ("Done?"=w43:bool)
      }
    }
    frame #2 {
      n149 = call <vilib>:"High Resolution Relative Seconds.vi"() -> ("relative seconds"=w349:dbl)
      n150 = Subtract(x=w349, y=w348) -> (x-y=w347:dbl)
    }
  }
  "runTime(s)" <- w1
